vi "Load.vi"(8 "error in (no error)":errorcluster, 11 "MusicLibrary in":refnum<class "MusicLibrary.lvclass">) -> (0 "error out":errorcluster, 3 "MusicLibrary out":refnum<class "MusicLibrary.lvclass">)   [LabVIEW 2015, in "MusicLibrary.lvclass"]
uses:
  MusicLibrary.lvclass
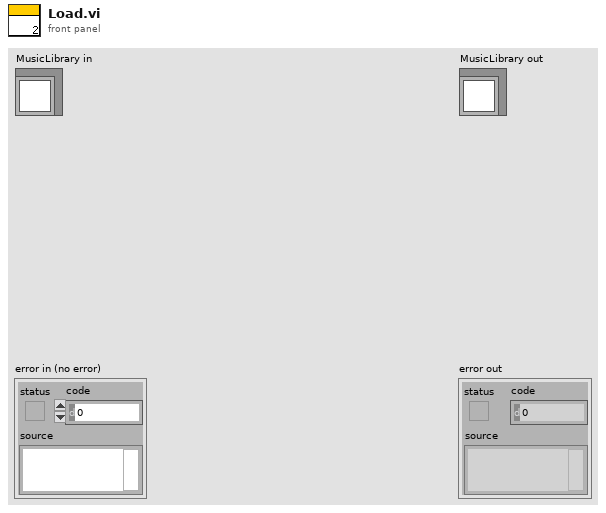
[diagram p1: front panel]
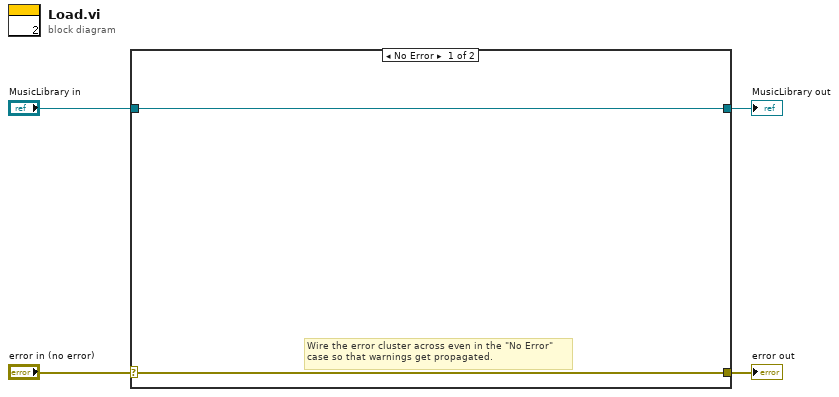
[diagram p0: block diagram]
diagram:
  n1 = case shown="No Error" "error in (no error)" {
    selector: "error in (no error)" -> [w5 w8]
    tunnel: [w5 w8] -> w3
    tunnel: [w6 w7] -> w1
    tunnel: "MusicLibrary in" -> [w6 w7]
    frame No Error {
      # "Wire the error cluster across even in the \"No Error\"\ncase so that warnings get propagated."
    }
    frame Error {
    }
  }
  "error out" <- w3
  "MusicLibrary out" <- w1
